vi "main02.vi"() -> ()   [LabVIEW 2018]
panel:
  out "Array":dbl[](array[numeric])
  in  "Anzahl Stützpunkte":dbl
  in  "Bottom":dbl
  in  "Top":dbl
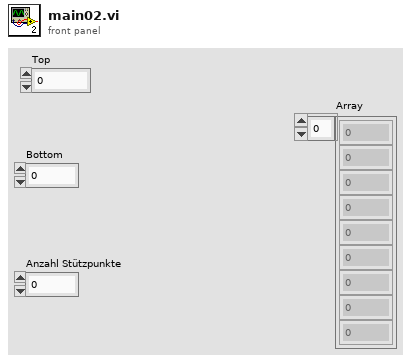
[diagram p1: front panel]
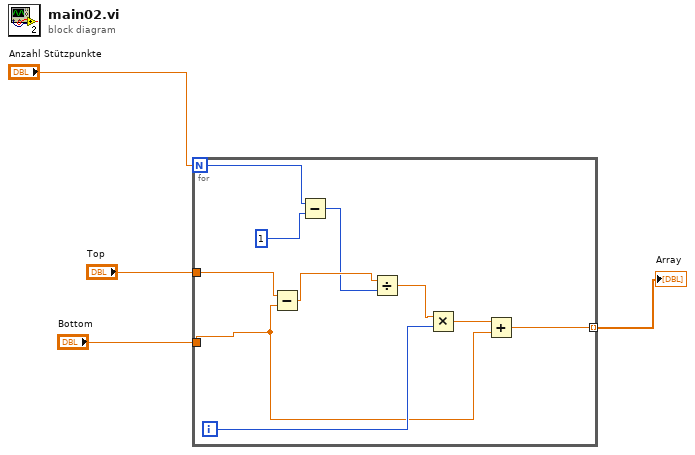
[diagram p0: block diagram]
diagram:
  n1 = for {
    N: "Anzahl Stützpunkte" -> [w14]
    tunnel: "Top" -> [w12]
    tunnel: "Bottom" -> [w5]
    tunnel: [w6] -> w1 mode=indexing
    i -> [w10]
    n2 = Subtract(x=w12, y=w5) -> (x-y=w9:dbl)
    n3 = Subtract(x=w14, y=1) -> (x-y=w8:i32)
    n4 = Divide(x=w9, y=w8) -> (x/y=w11:dbl)
    n5 = Multiply(x=w11, y=w10) -> (x*y=w7:dbl)
    n6 = Add(x=w7, y=w5) -> (x+y=w6:dbl)
  }
  "Array" <- w1
